vi "LCR Meter BIN Measurement.vi"() -> ()   [LabVIEW 2021, in "LCR Meter.lvlib"]
doc: "This example is simple BIN measurement."
uses:
  LCR Meter.lvlib
panel:
  out "Boolean":bool
  in  "stop":bool
  out "Comparator Result":string
  out "Secondary Value":dbl
  out "Primary Value":dbl
  in  "Serial Settings:Baud Rate":u32(ring)=115200 items=["9600"=9600, "38400"=38400, "57600"=57600, "115200"=115200]
  in  "VISA resource name":refnum<visa-resource-name>
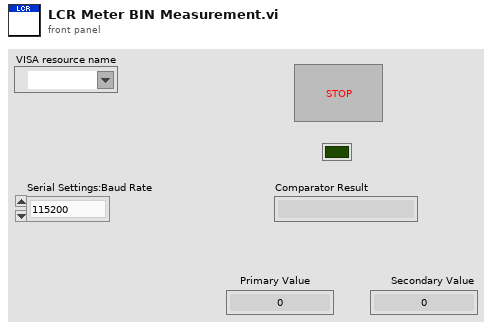
[diagram p1: front panel]
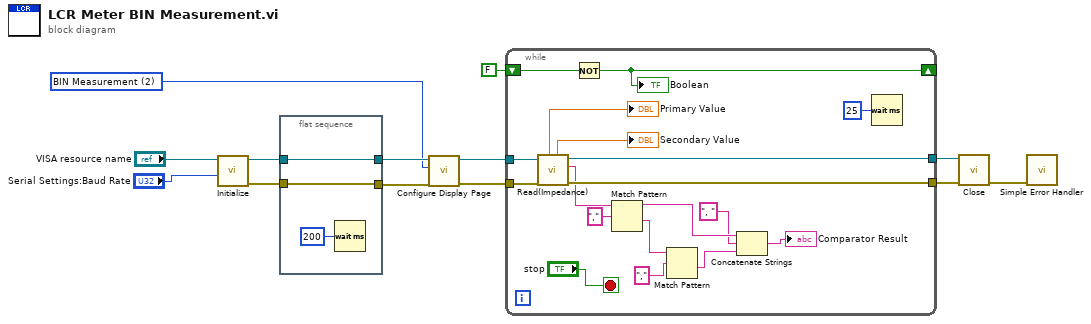
[diagram p0: block diagram]
diagram:
  w7 = u16 2 items=["Measurement", "Measurement Setup", "BIN Measurement", "BIN Count", "BIN Setup", "LIST Measurement", "LIST Setup", "CORRECTION", "CATALOG", "ENLARGE", "System Config", "System Information"] ("Display Page")
  n1 = call "Initialize.vi"("Serial Settings:Baud Rate"="Serial Settings:Baud Rate", "VISA resource name"="VISA resource name") -> ("error out"=w9:errorcluster, "VISA resource name out"=w11:refnum<visa-resource-name>)  [unwired: 7 in, 1 out]
  n2 = flat-sequence {
    tunnel: w11 -> [w16]
    tunnel: [w16] -> w10
    tunnel: [w15] -> w8
    tunnel: w9 -> [w15]
    frame #0 {
      n3 = Wait (ms)(milliseconds to wait=u32 200) -> ()  [unwired: 1 out]
    }
  }
  n4 = call "Configure Display Page.vi"("error in"=w8, "Display Page"=w7, "VISA resource name"=w10) -> ("error out"=w5:errorcluster, "VISA resource name out"=w6:refnum<visa-resource-name>)  [unwired: 7 in]
  n5 = while {
    tunnel: w6 -> [w34]
    tunnel: w5 -> [w33]
    tunnel: [w30] -> w3
    tunnel: [w29] -> w2
    shift-right: [w25] -> _
    shift-left: FALSE -> [w26]
    stop <- "stop" stop-if-true
    n6 = call "Read(Impedance).vi"("error in (no error)"=w33, "VISA resource name"=w34) -> ("error out"=w29:errorcluster, "Comparator Result"=w24:string, "VISA resource name out"=w30:refnum<visa-resource-name>, "Secondary Value"=→"Secondary Value":dbl, "Primary Value"=→"Primary Value":dbl)  [unwired: 3 in, 2 out]
    n7 = Not(x=w26) -> (.not. x?=w25:bool)
    "Boolean" <- w25
    n8 = Match Pattern(string=w24, regular expression=",") -> (before substring=w19:string, after substring=w22:string)  [unwired: 1 in, 2 out]
    n9 = Match Pattern(string=w22, regular expression=",") -> (after substring=w17:string)  [unwired: 1 in, 3 out]
    n10 = Concatenate Strings(w19, ", " ("string"), w17) -> (→"Comparator Result":string)
    n11 = Wait (ms)(milliseconds to wait=u32 25) -> ()  [unwired: 1 out]
  }
  n12 = call "Close.vi"("error in (no error)"=w2, "VISA resource name"=w3) -> ("error out"=w4:errorcluster)  [unwired: 9 in]
  n13 = call <vilib>:"Simple Error Handler.vi"("error in (no error)"=w4) -> ()  [unwired: 4 in, 5 out]
